vi "file test.vi"() -> ()   [LabVIEW 2016]
panel:
  out "Tool Offsets":T1
  out "offset":T2
  in  "path":path
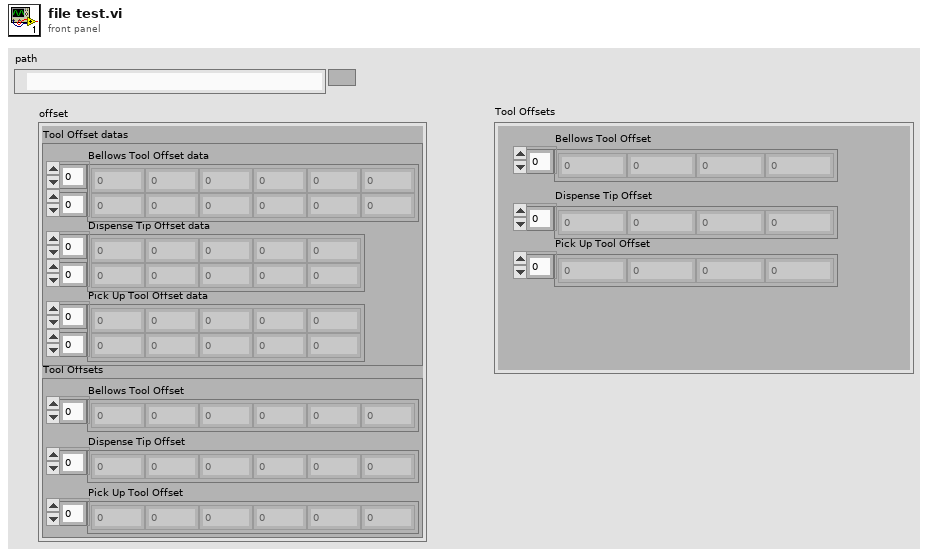
[diagram p1: front panel]
types:
  T1 = cluster{"Bellows Tool Offset":dbl[], "Dispense Tip Offset":dbl[], "Pick Up Tool Offset":dbl[]}
  T2 = cluster{"Tool Offset datas":cluster{"Bellows Tool Offset data":dbl[][], "Dispense Tip Offset data":dbl[][], "Pick Up Tool Offset data":dbl[][]}, "Tool Offsets":cluster{"Bellows Tool Offset":dbl[], "Dispense Tip Offset":dbl[], "Pick Up Tool Offset":dbl[]}}
  T3 = cluster{"controller":cluster{"A3200.lvclass":refnum<class "A3200.lvclass">, "Ultimus V2.lvclass":refnum<class "Ultimus V2.lvclass">, "NI-DAQ.lvclass":refnum<class "NI-DAQ.lvclass">}, "folder and file name":cluster{"Path":path, "folder name":string, "file name":string, "extension":string, "add time string":bool}, "IO":cluster{"Output num":dbl[], "Output ":bool[]}, "motion":cluster{"XYZU ":dbl[], "XY speed":dbl, "Z speed":dbl, "U speed":dbl}, "dispense":cluster{"Vacuum Setting (0000)":i64, "Pressure":i16, "on delay (ms)":dbl, "off delay (ms) ":dbl}}
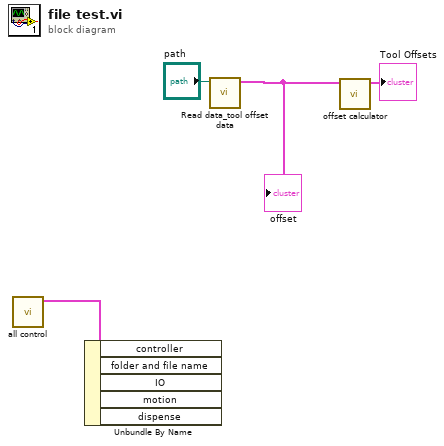
[diagram p0: block diagram]
diagram:
  n1 = call "all control.vi"() -> ("output cluster"=w1:T3)  [unwired: 11 in]
  n2 = Unbundle By Name(w1) -> ()  [unwired: 5 out]
  n3 = call "Read data_tool offset data.vi"("path"="path") -> ("offset"=w4:T2)  [unwired: 10 in]
  "offset" <- w4
  n4 = call "offset calculator.vi"("offset"=w4) -> ("Tool Offsets"=→"Tool Offsets":T1)  [unwired: 10 in]
